vi "HIOKI PW3390 Conf Measure Item sub1.vi"(1 "Power Sum":T1) -> (0 "Power Sum out":bool[][](array[boolean]))   [LabVIEW 2009]
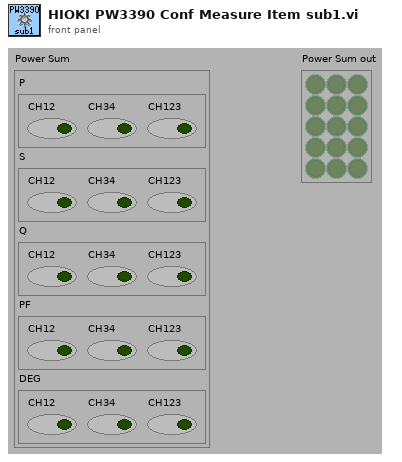
[diagram p1: front panel]
types:
  T1 = cluster{"P":cluster{"CH12":bool, "CH34":bool, "CH123":bool}, "S":cluster{"CH12":bool, "CH34":bool, "CH123":bool}, "Q":cluster{"CH12":bool, "CH34":bool, "CH123":bool}, "PF":cluster{"CH12":bool, "CH34":bool, "CH123":bool}, "DEG":cluster{"CH12":bool, "CH34":bool, "CH123":bool}}
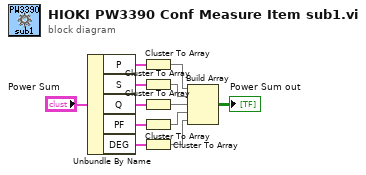
[diagram p0: block diagram]
diagram:
  n1 = Unbundle By Name("Power Sum") -> ("P"=w2:cluster{"CH12":bool, "CH34":bool, "CH123":bool}, "S"=w3:cluster{"CH12":bool, "CH34":bool, "CH123":bool}, "Q"=w4:cluster{"CH12":bool, "CH34":bool, "CH123":bool}, "PF"=w5:cluster{"CH12":bool, "CH34":bool, "CH123":bool}, "DEG"=w6:cluster{"CH12":bool, "CH34":bool, "CH123":bool})
  n2 = Cluster To Array(cluster=w2) -> (array=w7:bool[])
  n3 = Cluster To Array(cluster=w3) -> (array=w8:bool[])
  n4 = Cluster To Array(cluster=w4) -> (array=w9:bool[])
  n5 = Cluster To Array(cluster=w5) -> (array=w10:bool[])
  n6 = Cluster To Array(cluster=w6) -> (array=w11:bool[])
  n7 = Build Array(w7, w8, w9, w10, w11) -> (→"Power Sum out":bool[][])
